vi "SetGrabberPosition.vi"(8 "error in (no error)":errorcluster, 10 "GrabberPosition":dbl, 11 "JKI.Robot":refnum<class "JKI.Robot.SMO.lvclass">) -> (0 "error out":errorcluster, 3 "JKI.Robot out":refnum<class "JKI.Robot.SMO.lvclass">)   [LabVIEW 2014, in "JKI.Robot.SMO.lvclass"]
doc: "---------------------------------------------------------------\nJKI State Machine Objects™\nhttp://jki.net/state-machine-objects/\nCopyright (C) 2005-2015, JKI <info@jki.net>\nALL RIGHTS RESERVEDJKI State Machine Objects (SMO) 1.0.0.4\nJKI - JKI\nCopyright (c) 2015, JKI"
uses:
  JKI.Robot.SMO.lvclass
  JKI.Robot.SMO.lvclass/JKI.Robot.SMO.ctl
panel:
  # "For instructions on how to use the JKI State Machine Objects, examples and video tutorials, visit:\nhttp://jki.net/state-machine-objects/\n\nJKI State Machine Objects™\nhttp://jki.net/state-machine-objects/\nCopyright (C) 2005-2015, JKI <info@jki.net>\nALL RIGHTS RESERVED"
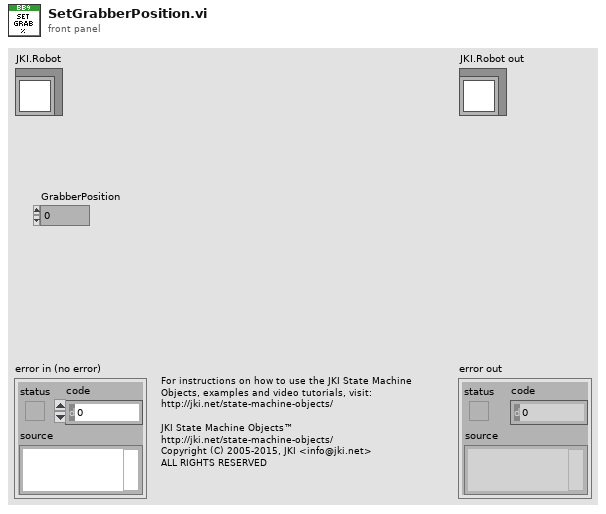
[diagram p1: front panel]
types:
  T1 = typedef "JKI.Robot.SMO.lvclass/PrivateData--Ref.ctl" = refnum<data-value>
  T2 = typedef "JKI.Robot.SMO.lvclass/PrivateData--Cluster.ctl" = cluster{"Configuration":T3, "Public Events":T4, "Robot Position":T5, "Private Events":T6}
  T3 = typedef "JKI.Robot.SMO.lvclass/Configuration--Cluster.ctl" = cluster{"Suffix":string}
  T4 = typedef "JKI.Robot.SMO.lvclass/PublicEvents--Cluster.ctl" = cluster{"Data Changed":refnum<user-event>}
  T5 = typedef "RobotPosition--Cluster.ctl" = cluster{"Claw%":dbl, "JointA":dbl, "JointB":dbl, "JointC":dbl}
  T6 = typedef "JKI.Robot.SMO.lvclass/PrivateEvents--Cluster.ctl" = cluster{"SetGrabberPosition":refnum<user-event>, "SetJointRotation":refnum<user-event>}
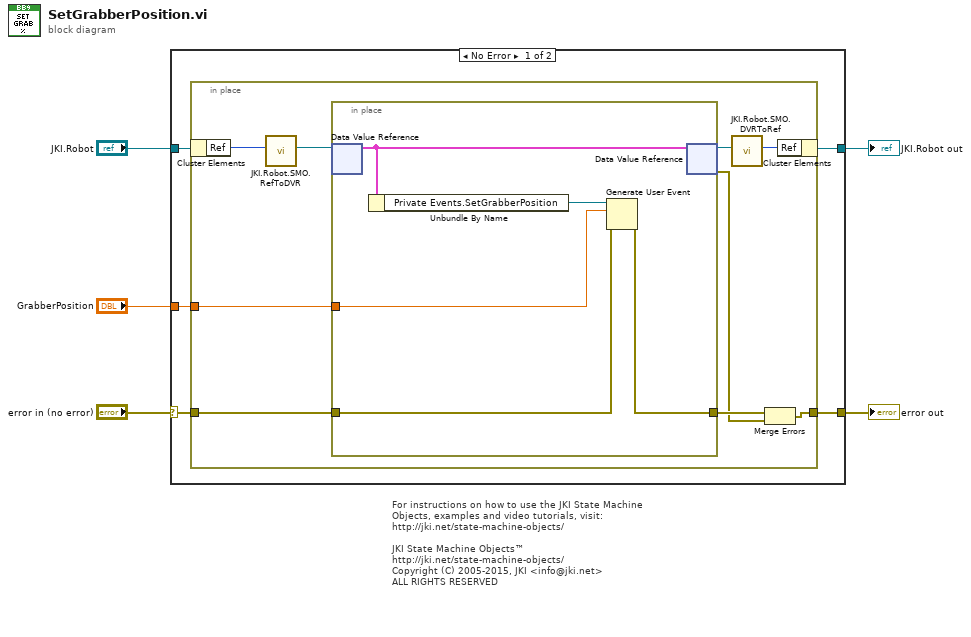
[diagram p0: block diagram]
diagram:
  # "For instructions on how to use the JKI State Machine Objects, examples and video tutorials, visit:\nhttp://jki.net/state-machine-objects/\n\nJKI State Machine Objects™\nhttp://jki.net/state-machine-objects/\nCopyright (C) 2005-2015, JKI <info@jki.net>\nALL RIGHTS RESERVED"
  n1 = case shown="No Error" "error in (no error)" {
    selector: "error in (no error)" -> [w8 w26]
    tunnel: [w7 w26] -> w4
    tunnel: [w9 w25] -> w5
    tunnel: "JKI.Robot" -> [w10 w25]
    tunnel: "GrabberPosition" -> [w6 _]
    frame No Error {
      n2 = in-place {
        in-place-border: w8 -> [w19]
        in-place-border: [w16] -> w7
        in-place-border: w6 -> [w13]
        n3 = in-place-cluster #1(w10) -> ("Ref"=w15:u32)
        n4 = call "JKI.Robot.SMO.RefToDVR.vi"("Ref"=w15) -> ("Ref"=w12:T1)  [unwired: 10 in]
        n5 = in-place {
          in-place-border: w19 -> [w22]
          in-place-border: [w21] -> w18
          in-place-border: w13 -> [w20]
          n6 = in-place-dvr #2(w12) -> (w24:T2)  [unwired: 1 out]
          n7 = Unbundle By Name(w24) -> ("Private Events.SetGrabberPosition"=w23:refnum<user-event>)
          n8 = Generate User Event(user event=w23, event data cluster=w20, error in=w22) -> (error out=w21:errorcluster)  [unwired: 1 in, 1 out]
          n9 = in-place-dvr #2(w24) -> (w14:T1, w17:errorcluster)
        }
        n10 = call "JKI.Robot.SMO.DVRToRef.vi"("Ref"=w14) -> ("Ref"=w11:u32)  [unwired: 10 in]
        n11 = Merge Errors(w18, w17) -> (w16:errorcluster)
        n12 = in-place-cluster #1("Ref"=w11) -> (w9:refnum<class "JKI.Robot.SMO.lvclass">)
      }
    }
    frame Error {
    }
  }
  "error out" <- w4
  "JKI.Robot out" <- w5
